vi "PH_ForceSensor.panel.vi"(0 "object ref":refnum<vi>, 5 "error in (no error)":errorcluster) -> (19 "error out":errorcluster)   [LabVIEW 2014, in "PH_ForceSensor.lvlib"]
doc: "By this VI a ross relais can be monitored and switched. \n\nThe indicators \"CLOSED\", \"OPEN\" and \"SWITCH STATE\" show the value of the Beckhoff-Tag: blue indicates bad tag status reference problems, darkgreen false and lightgreen on. If everything is working fine, \"CLOSED\" and \"SWITCH STATE\" should show the same value, while \"OPEN\" has the opposite value. \n\nThe oval button switches the ross relais. It should be in the same state as the \"SWITCH STATE\" indicator. \n\n\"EXIT\" closes the front panel (GUI), while \"Delete Instance\" disconnects and removes the instance from the PCS.\n\nThis VI has no machine safety relevant logig: there is neither a check of internal conclict nor with other objects, for example conflict with other ross relais. Therefore it must be handled with care and should be operated by well educated operators only. It is forseen exclusively for direct operating and testing of the system. \n\nLicense Agreement for this software:\n\nCopyright (C)\nGesellschaft für Schwerionenforschung, GSI\nPlanckstr. 1\n64291 Darmstadt\nGermany\n\nContact: D.Beck@gsi.de \n\nThis program is free software; you can redistribute it and/or modify it under the terms of the GNU General Public License as published by the Free Software Foundation; either version 2 of the license, or (at your option) any later version.\n\nThis program is distributed in the hope that it will be useful, but WITHOUT ANYW ARRANTY; without even the implied warranty of MERCHANTABILITY or FITNESS FOR A PARTICULAR PURPOSE. See the GNU General License for more details (http://www.gnu.org).\n\nGesellschaft für Schwerionenforschung, GSI\nPlanckstr. 1, 64291 Darmstadt, Germany\nFor all questions and ideas contact: M.Richter@gsi.de, H.Brand@gsi.de or D.Beck@gsi.de.\nLast update: 18-DEC-2002"
uses:
  PH_ForceSensor.lvlib
  PH_StatusHandler/PH_StatusHandler.GUI element.ctl
  PH_ForceSensor.Dataset.ctl
  PH_ForceSensor.Ranges.ctl
  PH_ForceSensor.GUI Refs.ctl
  PH_BeamlineInformation/PH_BeamlineInformation.GUI Ref.ctl
  PH_Beamline_Chief/PH_Beamline_Chief.Section.ctl
  PH_BeamlineInformation/PH_BeamlineInformation.Powermeter.ctl
  PH_BeamlineInformation/PH_BeamlineInformation.Efficiency.ctl
  PH_SystemInformation/PH_SystemInformation.GUI Refs.ctl
  CSCore/CSObj/CSObj.lvlib
  PH_Common/PH_Common.lvlib
  PH_PSDBWriter/PH_PSDBWriter.lvlib
  PH_Class/PH_Class.lvlib
  CSCore/CSSystem/CSSystemLib/CSSystemLib.lvlib
  PH_BeamlineInformation/PH_BeamlineInformation.lvlib
  PH_Beamline_Chief/PH_Beamline_Chief.lvlib
  PH_SystemInformation/PH_SystemInformation.lvlib
  PH_StatusHandler/PH_StatusHandler.lvlib
panel:
  in  "Tab Control":T1(tab)
  out "Voltage MA 5":dbl caption="[V]"
  out "Voltage MA 4":dbl caption="[V]"
  out "Voltage MA 3":dbl caption="[V]"
  out "Voltage MA 2":dbl caption="[V]"
  out "Voltage MA 1":dbl caption="[V]"
  out "PU MA 5":bool caption="State PU"
  out "PU MA 4":bool caption="State PU"
  out "PU MA 3":bool caption="State PU"
  out "PU MA 2":bool caption="State PU"
  out "PU MA 1":bool caption="State PU"
  out "Graph Differential Forces":cluster{dbl, dbl}(graph)={0.8278603788500902, 1.2559723352693055} caption="Differential Forces"
  in  "Ranges [N]":T2
  out "Graph Absolute Forces":cluster{dbl, dbl, dbl, dbl}(graph)={110.26863084922009, 111.09649122807018, 111.51252408477845, 112.76849642004775} caption="Absolute Forces"
  out "Rawvalues":T3
  in  "Offsets [µV]":T3
  out "Sensor Values [µV]":T3
  out "Forces [N]":T3
  in  "Scalings [mV/V]":T3
  in  "Supply Voltage [V]":dbl
  in  "Full Force [N]":dbl
  out "PSDB Status":u32(colorbox)=6618880 caption="PSDB"
  out "Status":T4 caption="Enabling State"
  in  "Delete":bool
  in  "Exit":bool
  out "loop counter":i32
  # "PCS"
  # "3.40"
  # "x"
  # "+"
  # "x"
  # ":"
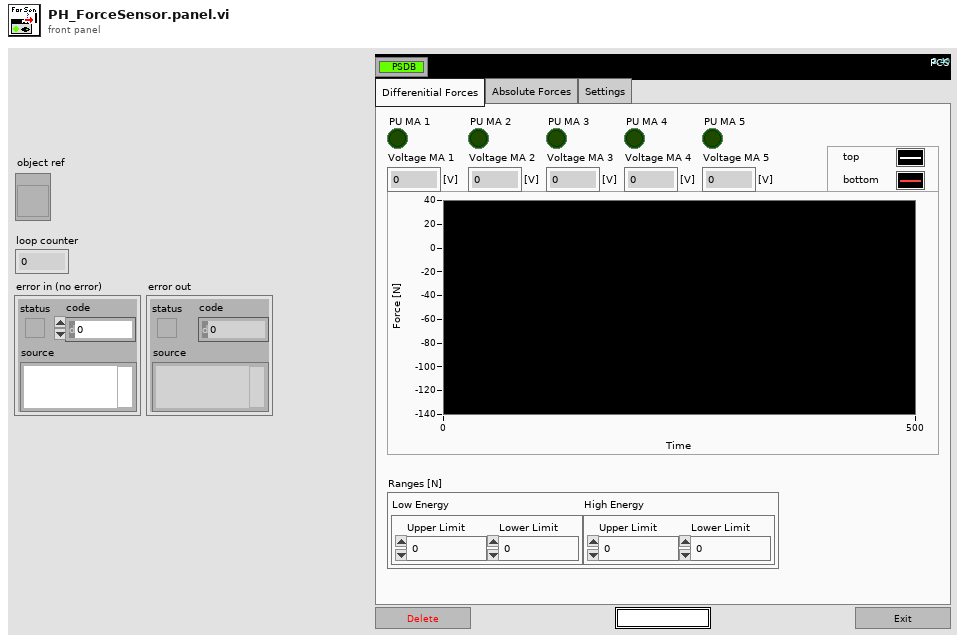
[diagram p1: front panel]
types:
  T1 = enum32{"Differenitial Forces", "Absolute Forces", "Settings"}
  T2 = typedef "PH_ForceSensor.lvlib/PH_ForceSensor.Ranges.ctl" = cluster{"Low Energy":cluster{"Upper Limit":dbl, "Lower Limit":dbl}, "High Energy":cluster{"Upper Limit":dbl, "Lower Limit":dbl}}
  T3 = typedef "PH_ForceSensor.lvlib/PH_ForceSensor.Dataset.ctl" = cluster{"top front":dbl, "top back":dbl, "bottom front":dbl, "bottom back":dbl}
  T4 = typedef "PH_StatusHandler.lvlib/PH_StatusHandler.GUI element.ctl" = u16
  T5 = typedef "PH_BeamlineInformation.lvlib/PH_BeamlineInformation.GUI Ref.ctl" = cluster{"BL Elements":cluster{"GUI Ref":refnum<vi>, "Beamline Section":T6}[], "Powermeters":T7, "Efficiency GUI Refs":T8, "Head GUI Refs":cluster{"PA - 19 - 1":cluster{"in Use":refnum<vi>, "voltage":refnum<vi>}, "PA - 19 - 2":cluster{"in Use":refnum<vi>, "voltage":refnum<vi>}, "PA - 45":cluster{"in Use":refnum<vi>, "voltage":refnum<vi>}, "PA - 45 - DP":cluster{"in Use":refnum<vi>, "voltage":refnum<vi>}, "MA - 1":cluster{"in Use":refnum<vi>, "voltage":refnum<vi>}, "MA - 2":cluster{"in Use":refnum<vi>, "voltage":refnum<vi>}, "MA - 3":cluster{"in Use":refnum<vi>, "voltage":refnum<vi>}, "MA - 4":cluster{"in Use":refnum<vi>, "voltage":refnum<vi>}, "MA - 5":cluster{"in Use":refnum<vi>, "voltage":refnum<vi>}, "MA - FR":cluster{"in Use":refnum<vi>, "voltage":refnum<vi>}}, "System Information GUI Refs":T9}
  T6 = typedef "PH_Beamline_Chief.lvlib/PH_Beamline_Chief.Section.ctl" = enum16{"None", "YLF", "fs", "fs-YLF", "ns", "PA-Input", "PA-Undelay", "PA-Delay", "PA-before-Bypass", "PA", "PA-Bypass", "PA-Exit", "PA-LL", "LL", "PA-MA", "MA-Exit", "MA-Z6", "Z6", "MA-LB", "LB-TB2", "LB-TB3"}
  T7 = typedef "PH_BeamlineInformation.lvlib/PH_BeamlineInformation.Powermeter.ctl" = cluster{"ns FE":cluster{"GUI Ref":refnum<vi>, "Value":dbl}, "fs FE":cluster{"GUI Ref":refnum<vi>, "Value":dbl}, "PA":cluster{"GUI Ref":refnum<vi>, "Value":dbl}, "MA":cluster{"GUI Ref":refnum<vi>, "Value":dbl}, "Z6 green":cluster{"GUI Ref":refnum<vi>, "Value":dbl}, "Z6 IR":cluster{"GUI Ref":refnum<vi>, "Value":dbl}, "Z6 COS":cluster{"GUI Ref":refnum<vi>, "Value":dbl}}
  T8 = typedef "PH_BeamlineInformation.lvlib/PH_BeamlineInformation.Efficiency.ctl" = cluster{"PA Gain":cluster{"GUI Ref":refnum<vi>, "Value":dbl}, "MA Gain":cluster{"GUI Ref":refnum<vi>, "Value":dbl}, "Z6 green Conversion":cluster{"GUI Ref":refnum<vi>, "Value":dbl}, "Z6 Comp Losses":cluster{"GUI Ref":refnum<vi>, "Value":dbl}}
  T9 = typedef "PH_SystemInformation.lvlib/PH_SystemInformation.GUI Refs.ctl" = cluster{"Laser":refnum<vi>, "PreAmp":refnum<vi>, "MainAmp":refnum<vi>, "Emergency Off":refnum<vi>, "Exp 1":refnum<vi>, "Exp 2":refnum<vi>, "Exp 3":refnum<vi>, "Exp 4":refnum<vi>, "Timing Mode GUI Ref":refnum<vi>}
  T10 = typedef "PH_ForceSensor.lvlib/PH_ForceSensor.GUI Refs.ctl" = cluster{"Delete":refnum<vi>, "Rawvalues":refnum<vi>, "Offsets [µV]":refnum<vi>, "Sensor Values [µV]":refnum<vi>, "Scalings [mV/V]":refnum<vi>, "Supply Voltage [V]":refnum<vi>, "Full Force [N]":refnum<vi>, "Forces [N]":refnum<vi>, "Graph Differential Forces":refnum<vi>, "Graph Absolute Forces":refnum<vi>, "Ranges [N]":refnum<vi>}
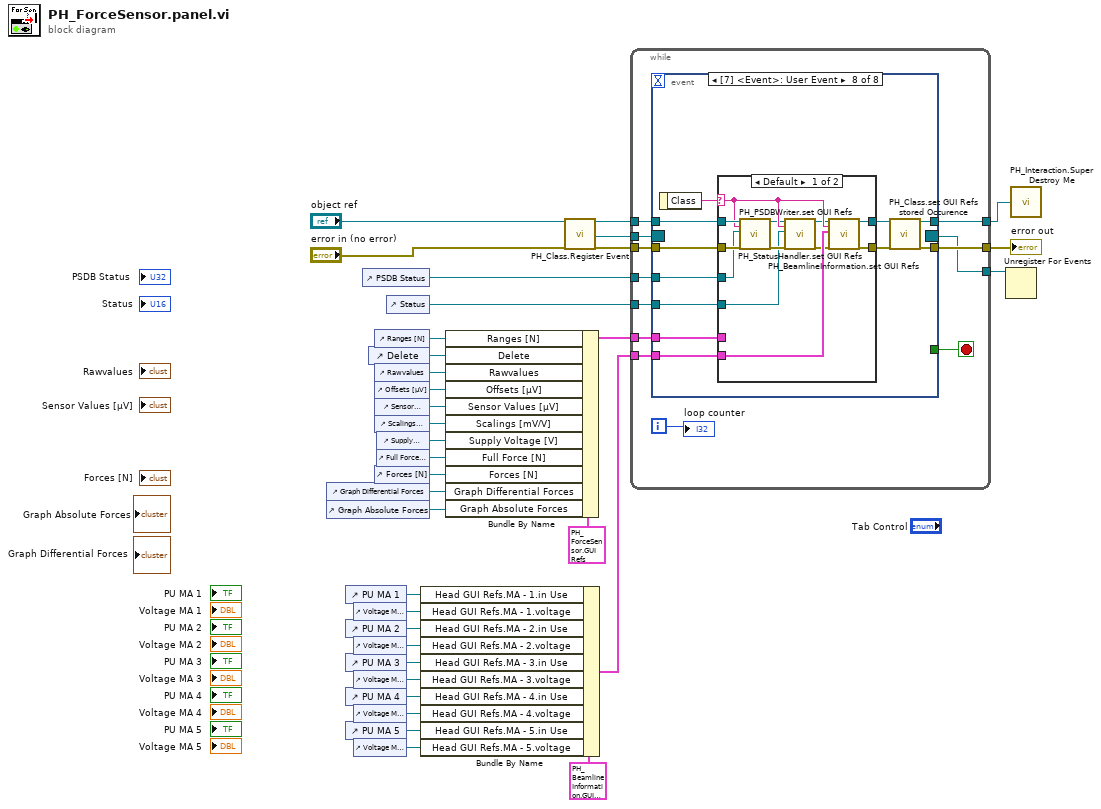
[diagram p0: block diagram]
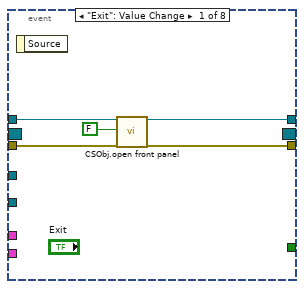
[diagram p2: hidden frame]
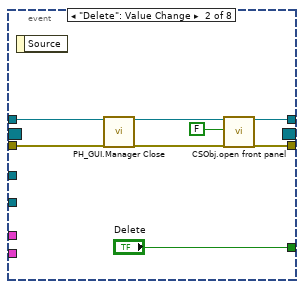
[diagram p3: hidden frame]
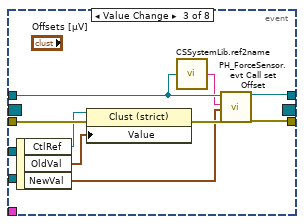
[diagram p4: hidden frame]
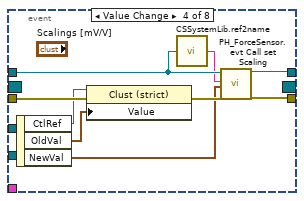
[diagram p5: hidden frame]
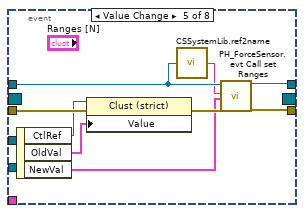
[diagram p6: hidden frame]
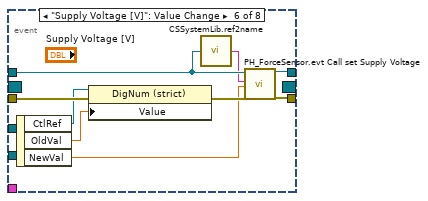
[diagram p7: hidden frame]
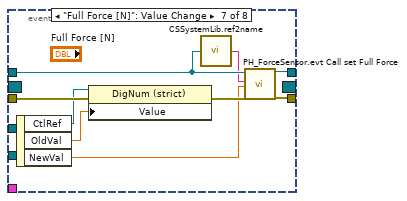
[diagram p8: hidden frame]
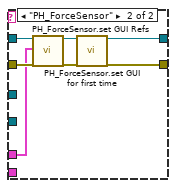
[diagram p9: hidden frame]
diagram:
  n1 = control-ref of="Graph Differential Forces"() -> (w16:refnum<vi>)
  n2 = control-ref of="Graph Absolute Forces"() -> (w15:refnum<vi>)
  n3 = control-ref of="PU MA 1"() -> (w13:refnum<vi>)
  n4 = control-ref of="PU MA 2"() -> (w11:refnum<vi>)
  n5 = control-ref of="PU MA 3"() -> (w9:refnum<vi>)
  n6 = control-ref of="PU MA 4"() -> (w7:refnum<vi>)
  n7 = control-ref of="PU MA 5"() -> (w5:refnum<vi>)
  n8 = control-ref of="Voltage MA 1"() -> (w12:refnum<vi>)
  n9 = control-ref of="Voltage MA 2"() -> (w10:refnum<vi>)
  n10 = control-ref of="Voltage MA 3"() -> (w8:refnum<vi>)
  n11 = control-ref of="Voltage MA 4"() -> (w6:refnum<vi>)
  n12 = control-ref of="Voltage MA 5"() -> (w4:refnum<vi>)
  n13 = control-ref of="PSDB Status"() -> (w29:refnum<vi>)
  n14 = control-ref of="Delete"() -> (w35:refnum<vi>)
  n15 = control-ref of="Ranges [N]"() -> (w2:refnum<vi>)
  n16 = control-ref of="Rawvalues"() -> (w23:refnum<vi>)
  n17 = control-ref of="Offsets [µV]"() -> (w22:refnum<vi>)
  n18 = control-ref of="Sensor Values [µV]"() -> (w21:refnum<vi>)
  n19 = control-ref of="Scalings [mV/V]"() -> (w20:refnum<vi>)
  n20 = control-ref of="Forces [N]"() -> (w17:refnum<vi>)
  n21 = control-ref of="Supply Voltage [V]"() -> (w19:refnum<vi>)
  n22 = control-ref of="Full Force [N]"() -> (w18:refnum<vi>)
  n23 = control-ref of="Status"() -> (w1:refnum<vi>)
  n24 = Bundle By Name(cluster=T5 {"BL Elements"=[], "Powermeters"={"ns FE"={"GUI Ref"=refnum, "Value"=-1.0}, "fs FE"={"GUI Ref"=refnum, "Value"=-1.0}, "PA"={"GUI Ref"=refnum, "Value"=-1.0}, "MA"={"GUI Ref"=refnum, "Value"=-1.0}, "Z6 green"={"GUI Ref"=refnum, "Value"=-1.0}, "Z6 IR"={"GUI Ref"=refnum, "Value"=-1.0}, "Z6 COS"={"GUI Ref"=refnum, "Value"=-1.0}}, "Efficiency GUI Refs"={"PA Gain"={"GUI Ref"=refnum, "Value"=-1.0}, "MA Gain"={"GUI Ref"=refnum, "Value"=-1.0}, "Z6 green Conversion"={"GUI Ref"=refnum, "Value"=-1.0}, "Z6 Comp Losses"={"GUI Ref"=refnum, "Value"=-1.0}}, "Head GUI Refs"={"PA - 19 - 1"={"in Use"=refnum, "voltage"=refnum}, "PA - 19 - 2"={"in Use"=refnum, "voltage"=refnum}, "PA - 45"={"in Use"=refnum, "voltage"=refnum}, "PA - 45 - DP"={"in Use"=refnum, "voltage"=refnum}, "MA - 1"={"in Use"=refnum, "voltage"=refnum}, "MA - 2"={"in Use"=refnum, "voltage"=refnum}, "MA - 3"={"in Use"=refnum, "voltage"=refnum}, "MA - 4"={"in Use"=refnum, "voltage"=refnum}, "MA - 5"={"in Use"=refnum, "voltage"=refnum}, "MA - FR"={"in Use"=refnum, "voltage"=refnum}}, "System Information GUI Refs"={"Laser"=refnum, "PreAmp"=refnum, "MainAmp"=refnum, "Emergency Off"=refnum, "Exp 1"=refnum, "Exp 2"=refnum, "Exp 3"=refnum, "Exp 4"=refnum, "Timing Mode GUI Ref"=refnum}} ("BeamlineInformation GUI Refs"), "Head GUI Refs.MA - 1.in Use"=w13, "Head GUI Refs.MA - 1.voltage"=w12, "Head GUI Refs.MA - 2.in Use"=w11, "Head GUI Refs.MA - 2.voltage"=w10, "Head GUI Refs.MA - 3.in Use"=w9, "Head GUI Refs.MA - 3.voltage"=w8, "Head GUI Refs.MA - 4.in Use"=w7, "Head GUI Refs.MA - 4.voltage"=w6, "Head GUI Refs.MA - 5.in Use"=w5, "Head GUI Refs.MA - 5.voltage"=w4) -> (w3:T5)
  n25 = Bundle By Name(cluster=T10 {"Delete"=refnum, "Rawvalues"=refnum, "Offsets [µV]"=refnum, "Sensor Values [µV]"=refnum, "Scalings [mV/V]"=refnum, "Supply Voltage [V]"=refnum, "Full Force [N]"=refnum, "Forces [N]"=refnum, "Graph Differential Forces"=refnum, "Graph Absolute Forces"=refnum, "Ranges [N]"=refnum} ("GUI Refs"), "Ranges [N]"=w2, "Delete"=w35, "Rawvalues"=w23, "Offsets [µV]"=w22, "Sensor Values [µV]"=w21, "Scalings [mV/V]"=w20, "Supply Voltage [V]"=w19, "Full Force [N]"=w18, "Forces [N]"=w17, "Graph Differential Forces"=w16, "Graph Absolute Forces"=w15) -> (w24:T10)
  n26 = call "PH_Class.Register Event.vi"("i ref in"="object ref", "error in (no error)"="error in (no error)") -> ("i ref out"=w32:refnum<vi>, "Event Registration Refnum"=w30:refnum<event-registration>, "error out"=w31:errorcluster)  [unwired: 15 in]
  n27 = while {
    tunnel: w32 -> [w43]
    tunnel: [w42] -> w34
    tunnel: w31 -> [w45]
    tunnel: [w44] -> w33
    tunnel: w30 -> [w39]
    tunnel: w29 -> [w41]
    tunnel: [w38] -> w28
    tunnel: w24 -> [w40]
    tunnel: w3 -> [w37]
    tunnel: w1 -> [w36]
    i -> [w46]
    stop <- w47 stop-if-true
    n28 = event shown="[7] <Event>: User Event" {
      selector: w39 -> [_ _ _ _ _ _ _ _]
      dyn-events: [_ _ _ _ _ _ _ _] -> w38
      timeout: _ -> [_ _ _ _ _ _ _ _]
      tunnel: [_ "Delete" _ _ _ _ _ _] -> w47
      tunnel: w43 -> [w52 w54 w62 w71 w81 w90 w99 w116]
      tunnel: w45 -> [w50 w56 w69 w78 w87 w96 w105 w115]
      tunnel: [w49 w58 w65 w74 w83 w92 w101 w110] -> w44
      tunnel: [w48 w57 w64 w73 w82 w91 w100 w108] -> w42
      tunnel: w41 -> [_ _ _ _ _ _ _ w112]
      tunnel: w40 -> [_ _ _ _ _ _ _ w111]
      tunnel: w37 -> [_ _ _ _ _ _ _ w107]
      tunnel: w36 -> [_ _ _ _ _ _ _ w106]
      event "Exit": Value Change {
        n29 = event-data() -> ()  [unwired: 1 in, 1 out]
        n30 = call "CSObj.open front panel.vi"("i ref in"=w52, "frontPanelOpen"=FALSE ("front panel open"), "error in (no error)"=w50) -> ("i ref out"=w48:refnum<vi>, "error out"=w49:errorcluster)  [unwired: 15 in]
      }
      event "Delete": Value Change {
        n31 = event-data() -> ()  [unwired: 1 in, 1 out]
        n32 = call "PH_GUI.Manager Close.vi"("i ref in"=w54, "error in"=w56) -> ("i ref out"=w53:refnum<vi>, "error out"=w55:errorcluster)  [unwired: 16 in]
        n33 = call "CSObj.open front panel.vi"("i ref in"=w53, "frontPanelOpen"=FALSE ("front panel open"), "error in (no error)"=w55) -> ("i ref out"=w57:refnum<vi>, "error out"=w58:errorcluster)  [unwired: 15 in]
      }
      event Value Change {
        n34 = event-data() -> ("CtlRef"=w68:refnum<vi>, "OldVal"=w67:T3, "NewVal"=w63:T3)  [unwired: 1 in]
        n35 = property class="Clust (strict)"(reference=w68, error in=w69, "Value"=w67) -> (error out=w66:errorcluster)  [unwired: 1 out]
        n36 = call "CSSystemLib.ref2name.vi"("obj refnum"=w62) -> ("name"=w61:string)
        n37 = call "PH_ForceSensor.evt Call set Offset.vi"("i ref in"=w62, "Instance"=w61, "Offsets [µV]"=w63, "error in (no error)"=w66) -> ("i ref out"=w64:refnum<vi>, "error out"=w65:errorcluster)  [unwired: 14 in]
      }
      event Value Change {
        n38 = event-data() -> ("CtlRef"=w77:refnum<vi>, "OldVal"=w76:T3, "NewVal"=w72:T3)  [unwired: 1 in]
        n39 = property class="Clust (strict)"(reference=w77, error in=w78, "Value"=w76) -> (error out=w75:errorcluster)  [unwired: 1 out]
        n40 = call "CSSystemLib.ref2name.vi"("obj refnum"=w71) -> ("name"=w70:string)
        n41 = call "PH_ForceSensor.evt Call set Scaling.vi"("i ref in"=w71, "Instance"=w70, "Scalings [mV/V]"=w72, "error in (no error)"=w75) -> ("i ref out"=w73:refnum<vi>, "error out"=w74:errorcluster)  [unwired: 14 in]
      }
      event Value Change {
        n42 = event-data() -> ("CtlRef"=w86:refnum<vi>, "OldVal"=w85:T2, "NewVal"=w79:T2)  [unwired: 1 in]
        n43 = property class="Clust (strict)"(reference=w86, error in=w87, "Value"=w85) -> (error out=w84:errorcluster)  [unwired: 1 out]
        n44 = call "CSSystemLib.ref2name.vi"("obj refnum"=w81) -> ("name"=w80:string)
        n45 = call "PH_ForceSensor.evt Call set Ranges.vi"("i ref in"=w81, "Instance"=w80, "Ranges [N]"=w79, "error in (no error)"=w84) -> ("i ref out"=w82:refnum<vi>, "error out"=w83:errorcluster)  [unwired: 14 in]
      }
      event "Supply Voltage [V]": Value Change {
        n46 = event-data() -> ("CtlRef"=w95:refnum<vi>, "OldVal"=w94:dbl, "NewVal"=w88:dbl)  [unwired: 1 in]
        n47 = property class="DigNum (strict)"(reference=w95, error in=w96, "Value"=w94) -> (error out=w93:errorcluster)  [unwired: 1 out]
        n48 = call "CSSystemLib.ref2name.vi"("obj refnum"=w90) -> ("name"=w89:string)
        n49 = call "PH_ForceSensor.evt Call set Supply Voltage.vi"("i ref in"=w90, "Instance"=w89, "Supply Voltage [V]"=w88, "error in (no error)"=w93) -> ("i ref out"=w91:refnum<vi>, "error out"=w92:errorcluster)  [unwired: 14 in]
      }
      event "Full Force [N]": Value Change {
        n50 = event-data() -> ("CtlRef"=w104:refnum<vi>, "OldVal"=w103:dbl, "NewVal"=w97:dbl)  [unwired: 1 in]
        n51 = property class="DigNum (strict)"(reference=w104, error in=w105, "Value"=w103) -> (error out=w102:errorcluster)  [unwired: 1 out]
        n52 = call "CSSystemLib.ref2name.vi"("obj refnum"=w99) -> ("name"=w98:string)
        n53 = call "PH_ForceSensor.evt Call set Full Force.vi"("i ref in"=w99, "Instance"=w98, "Full Force [N]"=w97, "error in (no error)"=w102) -> ("i ref out"=w100:refnum<vi>, "error out"=w101:errorcluster)  [unwired: 14 in]
      }
      event User Event {
        n54 = event-data() -> ("Class"=w113:string)  [unwired: 1 in]
        n55 = case shown="Default" w113 {
          selector: w113 -> [w119 _]
          tunnel: w116 -> [w128 w135]
          tunnel: [w125 w129] -> w109
          tunnel: w115 -> [w127 w134]
          tunnel: [w123 w131] -> w114
          tunnel: w112 -> [w126 _]
          tunnel: w111 -> [_ w132]
          tunnel: w107 -> [w122 _]
          tunnel: w106 -> [w120 _]
          frame Default {
            n56 = call "PH_PSDBWriter.set GUI Refs.vi"("i ref in"=w128, "Class"=w119, "Ref PSDB Status"=w126, "error in"=w127) -> ("i ref out"=w118:refnum<vi>, "error out"=w124:errorcluster)  [unwired: 14 in]
            n57 = call "PH_StatusHandler.set GUI Refs.vi"("i ref in"=w118, "Class"=w119, "GUI Ref"=w120, "error in (no error)"=w124) -> ("i ref out"=w117:refnum<vi>, "error out"=w121:errorcluster)  [unwired: 14 in]
            n58 = call "PH_BeamlineInformation.set GUI Refs.vi"("Ref in"=w117, "Class"=w119, "BeamlineInformation GUI Refs"=w122, "error in"=w121) -> ("Ref out"=w125:refnum<vi>, "error out"=w123:errorcluster)  [unwired: 14 in]
          }
          frame "PH_ForceSensor" {
            n59 = call "PH_ForceSensor.set GUI Refs.vi"("VI in"=w135, "GUI Refs"=w132, "error in (no error)"=w134) -> ("VI out"=w130:refnum<vi>, "error out"=w133:errorcluster)  [unwired: 15 in]
            n60 = call "PH_ForceSensor.set GUI for first time.vi"("VI in"=w130, "error in (no error)"=w133) -> ("VI out"=w129:refnum<vi>, "error out"=w131:errorcluster)  [unwired: 16 in]
          }
        }
        n61 = call "PH_Class.set GUI Refs stored Occurence.vi"("i ref in"=w109, "error in (no error)"=w114) -> ("i ref out"=w108:refnum<vi>, "error out"=w110:errorcluster)  [unwired: 16 in]
      }
    }
    "loop counter" <- w46
  }
  "error out" <- w33
  n62 = Unregister For Events(event registration refnum=w28) -> ()  [unwired: 1 in, 1 out]
  n63 = call "PH_Interaction.Super Destroy Me.vi"("i ref out"=w34) -> ()
